vi "Example Debug Code 2.vi"() -> ()   [LabVIEW 2021]
uses:
  <userlib>/_OpenG.lib/string/string.llb/Convert EOLs (String)__ogtk.vi
panel:
  out "Array 2":i32[](array[numeric])
  out "sum":i32
  out "Array":string[](array[string])
  in  "Input":string="46threevqs8114\nthreetwoonez1gtrd\n6ffxbtff\n769twotwo6rv9\ngjrcjrkvghthreegqqrg82qbct\nzkxjhgprtrlcfeight795five8\n99seven3vdcgvmvxtjtwodc5\nthree5eightthree3four3vtkkqrgxs\nfour863mrrnrsxrkone\nsevenntgvnrrqfvxh2ttnkgffour8fiveone\n49fbsfb\n3rbmlsksg\nztgszqjjsrtmgqx6572\n3bqnfxkdbonesixseven\nmfgx32ftpbhgngm7\nfzrpfhbfvj6dbxbtfs7twofksfbshrzkdeightwoqg\n2xcftwo\ncshmmltsml4fiveeightdn\neightthsix1\ntwo1gvfxcqnrfnbeightthreexznhbmmk\n3917sevenvxqxntcgxskh\nksctcnfxdsk96drlbjkthreesfqlvnpvfbcbmg\n8nvrmzfs46\n5dbgltmgg1xvtqfkdxsrxzltwo1pgqlqndlc\neight7four6rpbtmjzj5\n41seven\ngpmfhninexxgqr6\n15sixdrhxzcmqf\n8fivettgmcs..."
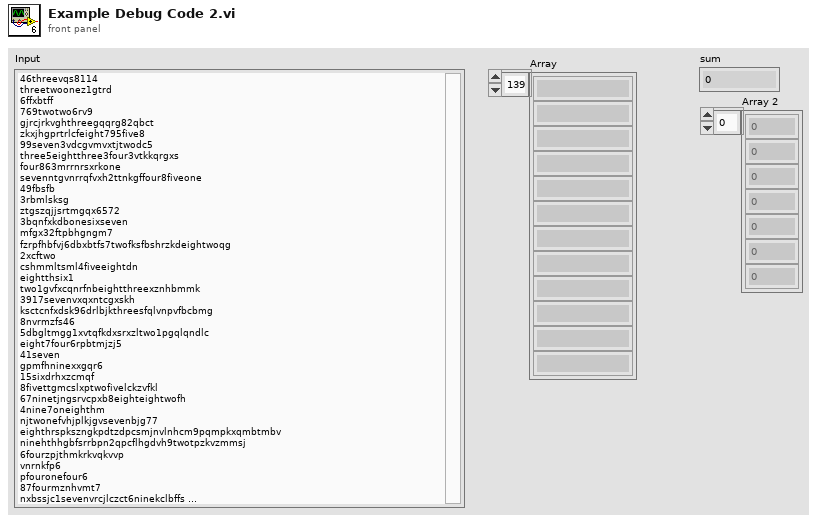
[diagram p1: front panel]
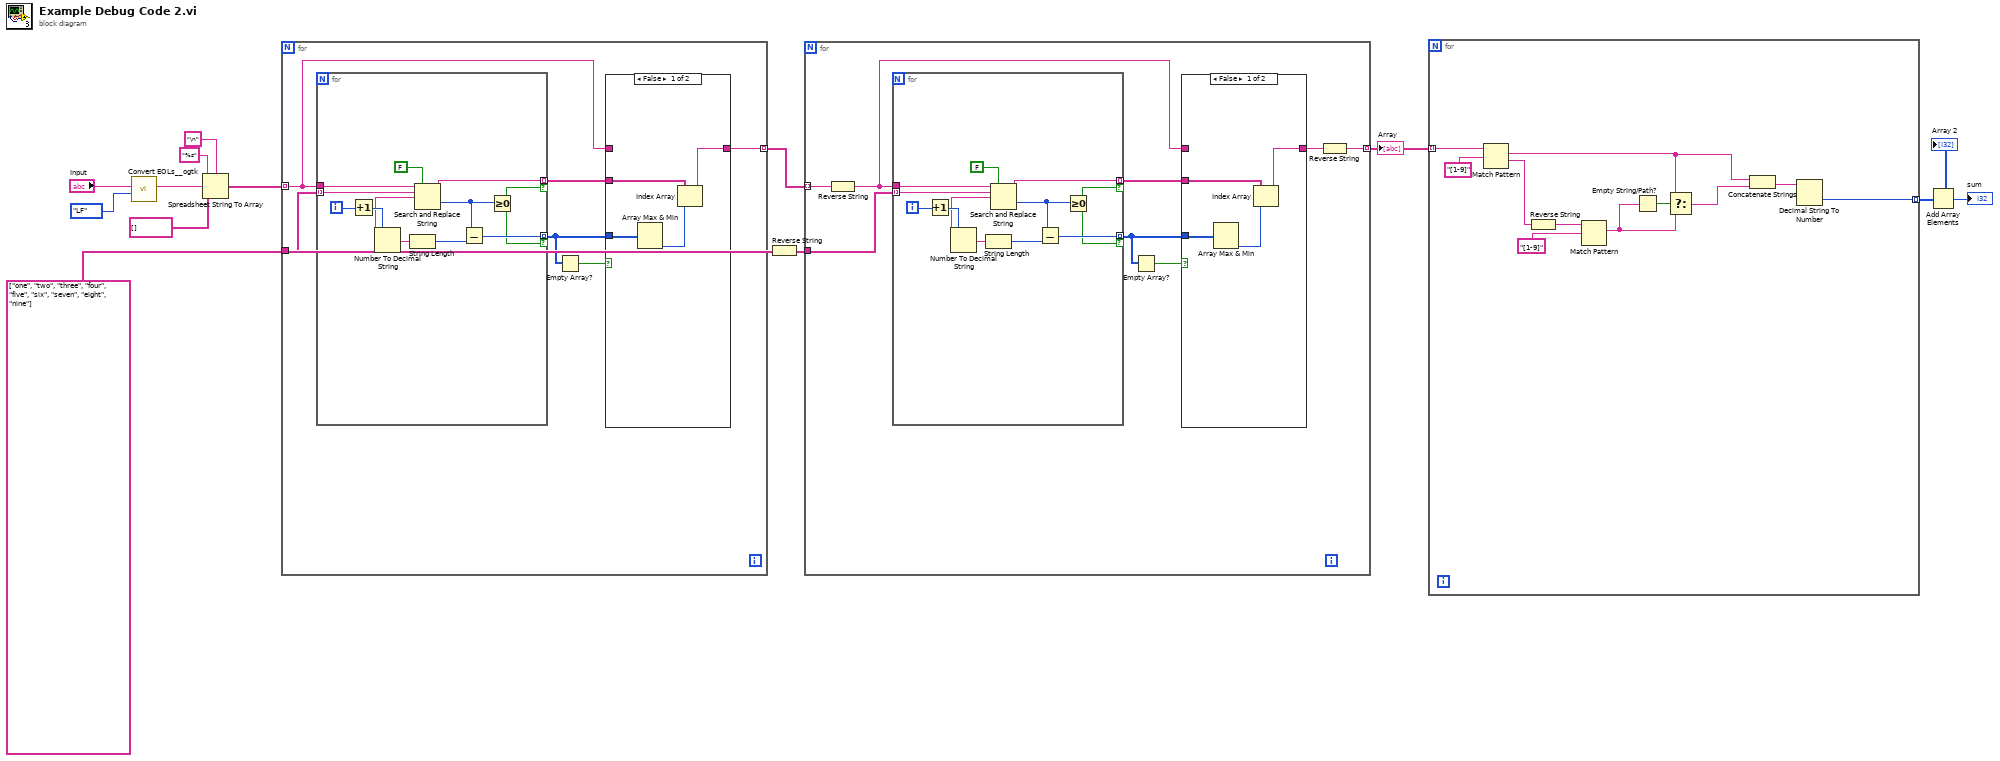
[diagram p0: block diagram]
diagram:
  w5 = string[] ["one", "two", "three", "four", "five", "six", "seven", "eight", "nine"]
  n1 = call-poly <userlib>:"Convert EOLs__ogtk.vi"("Convert to:"=enum16{"CR", "LF", "CRLF"}."LF", "String in"="Input") -> ("String out"=w9:string)  [unwired: 9 in]
  n2 = Spreadsheet String To Array(delimiter (Tab)="\n", format string="%s", spreadsheet string=w9, array type (2D Dbl)=string[] []) -> (array=w7:string[])
  n3 = for {
    tunnel: w7 -> [w17] mode=indexing
    tunnel: w5 -> [w19]
    tunnel: [w14] -> w6 mode=indexing
    n4 = for {
      tunnel: w17 -> [w35]
      tunnel: w19 -> [w33] mode=indexing
      tunnel: [w27] -> w16 mode=indexing if=w25
      tunnel: [w26] -> w15 mode=indexing if=w25
      i -> [w32]
      n5 = Increment(x=w32) -> (x+1=w31:i32)
      n6 = Number To Decimal String(number=w31) -> (decimal integer string=w30:string)  [unwired: 1 in]
      n7 = String Length(string=w30) -> (length=w29:i32)
      n8 = Search and Replace String(replace all?=FALSE, input string=w35, search string=w33, replace string=w30) -> (result string=w27:string, offset past replacement=w28:i32)  [unwired: 4 in, 2 out]
      n9 = Subtract(x=w28, y=w29) -> (x-y=w26:i32)
      n10 = Greater Or Equal To 0?(x=w28) -> (x >= 0?=w25:bool)
    }
    n11 = Empty Array?(array=w15) -> (empty?=w18:bool)
    n12 = case shown="False" w18 {
      tunnel: w17 -> [_ w24]
      tunnel: w16 -> [w22 _]
      tunnel: w15 -> [w23 _]
      tunnel: [w20 w24] -> w14
      frame False {
        n13 = Array Max & Min(array=w23) -> (min index (indices)=w21:i32)  [unwired: 3 out]
        n14 = Index Array(array=w22, index=w21) -> (element=w20:string)
      }
      frame True {
      }
    }
  }
  n15 = Reverse String(1:w5) -> (0:w4:string[])
  n16 = for {
    tunnel: w6 -> [w41] mode=indexing
    tunnel: w4 -> [w43]
    tunnel: [w36] -> w3 mode=indexing
    n17 = Reverse String(1:w41) -> (0:w37:string)
    n18 = for {
      tunnel: w37 -> [w59]
      tunnel: w43 -> [w57] mode=indexing
      tunnel: [w51] -> w40 mode=indexing if=w49
      tunnel: [w50] -> w39 mode=indexing if=w49
      i -> [w56]
      n19 = Increment(x=w56) -> (x+1=w55:i32)
      n20 = Number To Decimal String(number=w55) -> (decimal integer string=w54:string)  [unwired: 1 in]
      n21 = String Length(string=w54) -> (length=w53:i32)
      n22 = Search and Replace String(replace all?=FALSE, input string=w59, search string=w57, replace string=w54) -> (result string=w51:string, offset past replacement=w52:i32)  [unwired: 4 in, 2 out]
      n23 = Subtract(x=w52, y=w53) -> (x-y=w50:i32)
      n24 = Greater Or Equal To 0?(x=w52) -> (x >= 0?=w49:bool)
    }
    n25 = Empty Array?(array=w39) -> (empty?=w42:bool)
    n26 = case shown="False" w42 {
      tunnel: w37 -> [_ w48]
      tunnel: w40 -> [w46 _]
      tunnel: w39 -> [w47 _]
      tunnel: [w44 w48] -> w38
      frame False {
        n27 = Array Max & Min(array=w47) -> (min index (indices)=w45:i32)  [unwired: 3 out]
        n28 = Index Array(array=w46, index=w45) -> (element=w44:string)
      }
      frame True {
      }
    }
    n29 = Reverse String(1:w38) -> (0:w36:string)
  }
  "Array" <- w3
  n30 = for {
    tunnel: w3 -> [w70] mode=indexing
    tunnel: [w60] -> w2 mode=indexing
    n31 = Match Pattern(string=w70, regular expression="[1-9]") -> (match substring=w62:string, after substring=w67:string)  [unwired: 1 in, 2 out]
    n32 = Reverse String(1:w67) -> (0:w61:string)
    n33 = Match Pattern(string=w61, regular expression="[1-9]") -> (match substring=w63:string)  [unwired: 1 in, 3 out]
    n34 = Empty String/Path?(string/path=w63) -> (empty?=w64:bool)
    n35 = Select(t=w62, s=w64, f=w63) -> (s? t:f=w65:string)
    n36 = Concatenate Strings(w62, w65) -> (w66:string)
    n37 = Decimal String To Number(string=w66) -> (number=w60:i32)  [unwired: 2 in, 1 out]
  }
  "Array 2" <- w2
  n38 = Add Array Elements(numeric array=w2) -> (sum=→"sum":i32)
